vi "emitters to PDWs.vi"(8 "fs [Hz]":dbl=1.0 format="%.2f", 9 "end time":dbl[](array[numeric]), 10 "start time":dbl[](array[numeric]) format="%#_13g", 11 "emmiter":T1[](array[typedef])) -> (1 "my saturate":bool, 3 "sorted array":T2(array[cluster]))   [LabVIEW 2021]
uses:
  emitter params.ctl
  02974b87-4f9c-4a39-b6ec-6068b831107f.vi
  <vilib>/Comparison/Less/Less Functor/Less Functor.lvclass
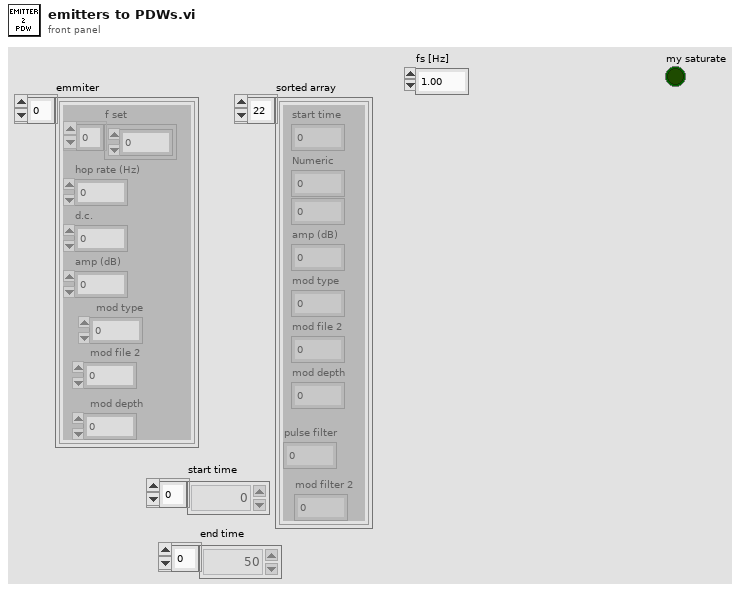
[diagram p1: front panel]
types:
  T1 = typedef "emitter params.ctl" = cluster{"f set":dbl[], "hop rate (Hz)":dbl, "d.c.":dbl, "amp (dB)":dbl, "mod type":u8, "mod file 2":u8, "mod depth":dbl}
  T2 = cluster{"start time":dbl, "Numeric":dbl, dbl, "amp (dB)":dbl, "mod type":u8, "mod file 2":u8, "mod depth":dbl, "pulse filter":u16, "mod filter 2":u16}[]
  T3 = cluster{"start time":dbl, "Numeric":dbl, dbl, dbl, "mod type":u8, "mod file 2":u8, "mod depth":dbl, u16, u16}
  T4 = cluster{"start time":dbl, "Numeric":dbl, dbl, dbl, "mod type":u8, "mod file 2":u8, "mod depth":dbl, u16, u16}[]
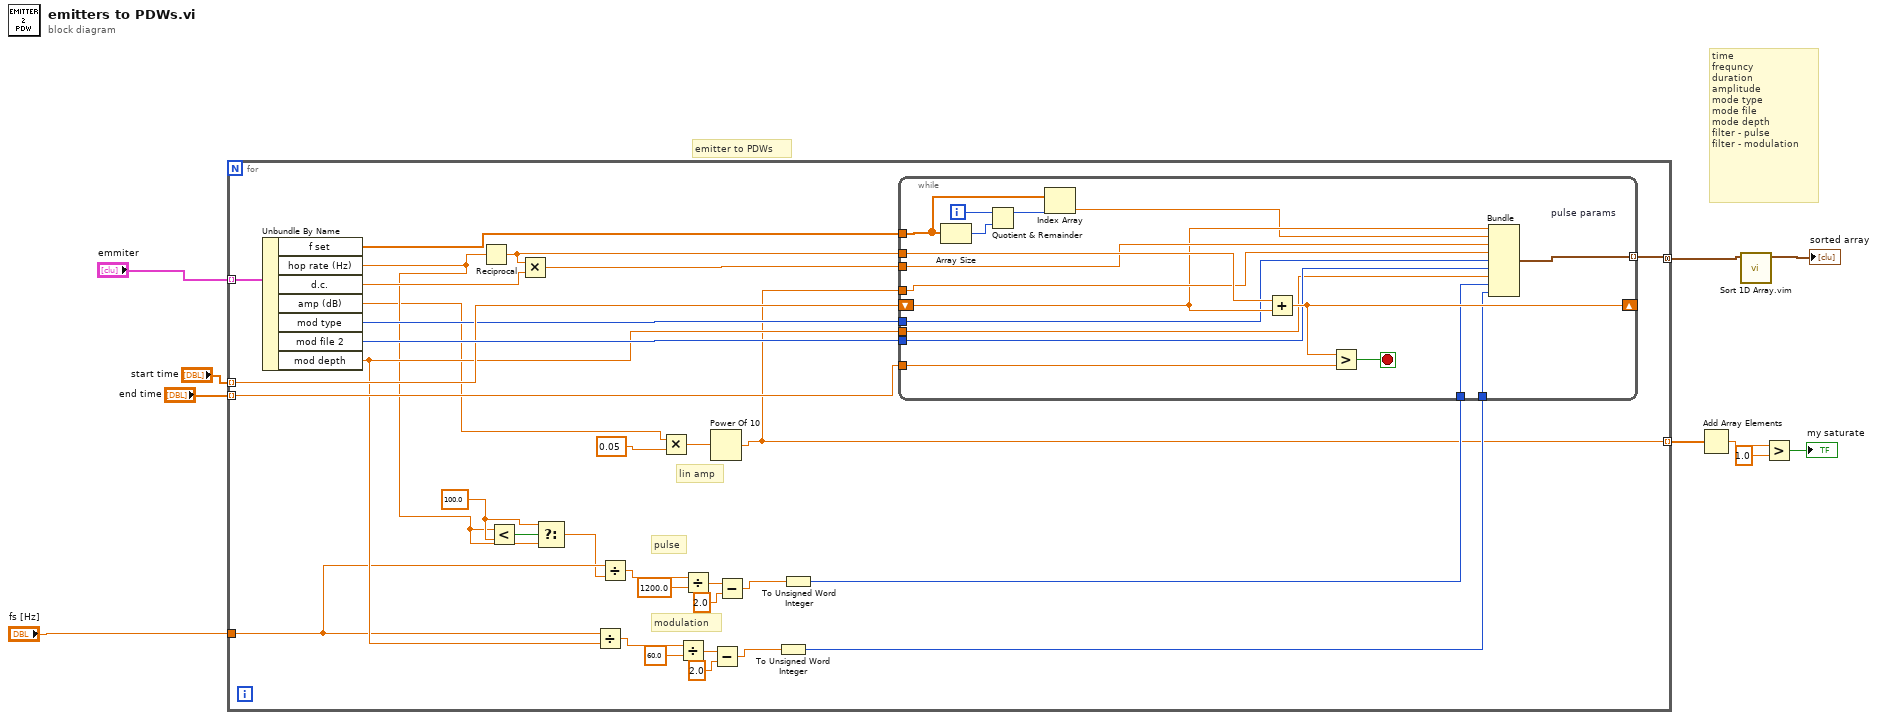
[diagram p0: block diagram]
diagram:
  # "time\nfrequncy\nduration\namplitude\nmode type\nmode file\nmode depth\nfilter - pulse\nfilter - modulation"
  # "emitter to PDWs"
  n1 = for {
    tunnel: "emmiter" -> [w42] mode=indexing
    tunnel: [w37] -> w9 mode=concatenating
    tunnel: "start time" -> [w35] mode=indexing
    tunnel: "end time" -> [w34] mode=indexing
    tunnel: "fs [Hz]" -> [w21]
    tunnel: [w11] -> w4 mode=indexing
    w17 = 100.0 ("y")
    # "lin amp"
    # "modulation"
    # "pulse"
    n2 = Unbundle By Name(w42) -> ("f set"=w41:dbl[], "hop rate (Hz)"=w15:dbl, "d.c."=w39:dbl, "amp (dB)"=w12:dbl, "mod type"=w33:u8, "mod file 2"=w36:u8, "mod depth"=w32:dbl)
    n3 = Reciprocal(x=w15) -> (1/x=w40:dbl)
    n4 = Less?(x=w15, y=w17) -> (x < y?=w18:bool)
    n5 = Multiply(x=w40, y=w39) -> (x*y=w38:dbl)
    n6 = Select(t=w17, s=w18, f=w15) -> (s? t:f=w16:dbl)
    n7 = Divide(x=w21, y=w32) -> (x/y=w31:dbl)
    n8 = Divide(x=w21, y=w16) -> (x/y=w22:dbl)
    n9 = Multiply(x=w12, y=0.05) -> (x*y=w13:dbl)
    n10 = Divide(x=w31, y=60.0) -> (x/y=w29:dbl)
    n11 = Divide(x=w22, y=1200.0) -> (x/y=w24:dbl)
    n12 = Power Of 10(x=w13) -> (10^x=w11:dbl)
    n13 = Subtract(x=w29, y=2.0) -> (x-y=w27:dbl)
    n14 = Subtract(x=w24, y=2.0) -> (x-y=w26:dbl)
    n15 = To Unsigned Word Integer(number=w27) -> (unsigned 16bit integer=w19:u16)
    n16 = To Unsigned Word Integer(number=w26) -> (unsigned 16bit integer=w20:u16)
    n17 = while {
      tunnel: w41 -> [w58]
      shift-right: [w54] -> _
      shift-left: w35 -> [w49]
      tunnel: w40 -> [w56]
      tunnel: w34 -> [w55]
      tunnel: w38 -> [w52]
      tunnel: w11 -> [w51]
      tunnel: [w50] -> w37 mode=indexing
      tunnel: w33 -> [w47]
      tunnel: w36 -> [w46]
      tunnel: w32 -> [w45]
      tunnel: w20 -> [w44]
      tunnel: w19 -> [w43]
      i -> [w60]
      stop <- w53 stop-if-true
      n18 = Array Size(array=w58) -> (size(s)=w59:i32)
      n19 = Quotient & Remainder(x=w60, y=w59) -> (x-y*floor(x/y)=w57:i32)  [unwired: 1 out]
      n20 = Index Array(array=w58, index=w57) -> (element=w48:dbl)
      n21 = Add(x=w56, y=w49) -> (x+y=w54:dbl)
      n22 = Greater?(x=w54, y=w55) -> (0:w53:bool)
      n23 = Bundle "pulse params"("start time"=w49, "Numeric"=w48, w52, w51, "mod type"=w47, "mod file 2"=w46, "mod depth"=w45, w44, w43) -> (w50:T3)  [unwired: 1 in]
    }
  }
  n24 = Add Array Elements(numeric array=w4) -> (sum=w3:dbl)
  n25 = call "Sort 1D Array.vim"("unsorted array"=w9) -> ("sorted array"=→"sorted array":T4)  [unwired: 10 in]
  n26 = Greater?(x=w3, y=1.0) -> (0:→"my saturate":bool)
